vi "Write Registers.vi"(6 "timeout ms (1000)":i32=1000, 8 "error in (no error)":errorcluster, 9 "Values":u16[](array[numeric]), 10 "Start Address":u16, 11 "TCP Network Connection in":refnum<k5>) -> (0 "error out":errorcluster, 3 "TCP Network Connection out":refnum<k5>)   [LabVIEW 2023, in "Modbus TCP Micro.lvlib"]
uses:
  Modbus TCP Micro.lvlib
  Modbus Functions.ctl
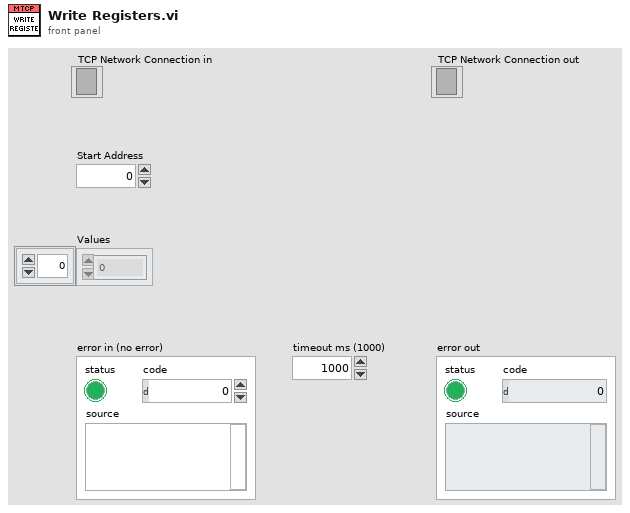
[diagram p1: front panel]
types:
  T1 = typedef "Modbus TCP Micro.lvlib/Modbus Functions.ctl" = u8
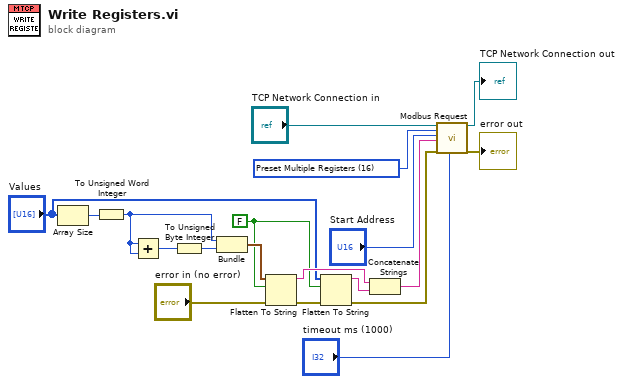
[diagram p0: block diagram]
diagram:
  w2 = T1 16 items=["None"=0, "Read Coil Status"=1, "Read Input Status"=2, "Read Holding Registers"=3, "Read Input Registers"=4, "Force Single Coil"=5, "Preset Single Register"=6, "Force Multiple Coils"=15, "Preset Multiple Registers"=16] ("Function Codes")
  w6 = FALSE ("prepend array or string size? (T)")
  n1 = Array Size(array="Values") -> (size(s)=w14:i32)
  n2 = To Unsigned Word Integer(number=w14) -> (unsigned 16bit integer=w13:u16)
  n3 = Add(x=w13, y=w13) -> (x+y=w12:u16)
  n4 = To Unsigned Byte Integer(number=w12) -> (unsigned 8bit integer=w11:u8)
  n5 = Bundle(w13, w11) -> (w10:cluster{u16, u8})  [unwired: 1 in]
  n6 = Flatten To String(anything=w10, prepend array or string size? (T)=w6, error in (no error)="error in (no error)") -> (data string=w15:string, error out=w5:errorcluster)  [unwired: 1 in, 1 out]
  n7 = Flatten To String(anything="Values", prepend array or string size? (T)=w6, error in (no error)=w5) -> (data string=w7:string, error out=w4:errorcluster)  [unwired: 1 in, 1 out]
  n8 = Concatenate Strings(w15, w7) -> (w8:string)
  n9 = call "Modbus Request.vi"("TCP Network Connection in"="TCP Network Connection in", "Function Codes"=w2, "Start Address"="Start Address", "Payload"=w8, "error in (no error)"=w4, "timeout ms (1000)"="timeout ms (1000)") -> ("TCP Network Connection out"=→"TCP Network Connection out":refnum<k5>, "error out"=→"error out":errorcluster)  [unwired: 8 in, 4 out]
